vi "TL behavior P-Wall.vi"(1 "Behavior\nVelocity":dbl=20.0, 2 "Activate?":bool=TRUE, 3 "Sensor":T1=[{"Name"="bow", "Angle"=20.0, "Distance"=0.0}, {"Name"="pbow", "Angle"=60.0, "Distance"=0.0}, {"Name"="port", "Angle"=0.0, "Distance"=0.0}, {"Name"="sbow", "Angle"=60.0, "Distance"=0.0}, {"Name"="starboard", "Angle"=0.0, "Distance"=0.0}]) -> (0 "P-Wall Array":dbl[](array[numeric]))   [LabVIEW 2014]
doc: "This vi creates a array based upon the value of the PBow IR sensor reading."
uses:
  sensorsSTD.ctl
  <vilib>/addons/control/pid/pid.llb/PID (DBL).vi
  <vilib>/addons/control/pid/NI_PID_pid.lvlib
panel:
  in  "setpoint":dbl=40.0 format="%#_13g"
  out "steer":dbl format="%.2f"
  out "Sensor \nbeing used":string
  out "Waveform Graph":cluster{dbl, dbl, dbl[]}(graph)
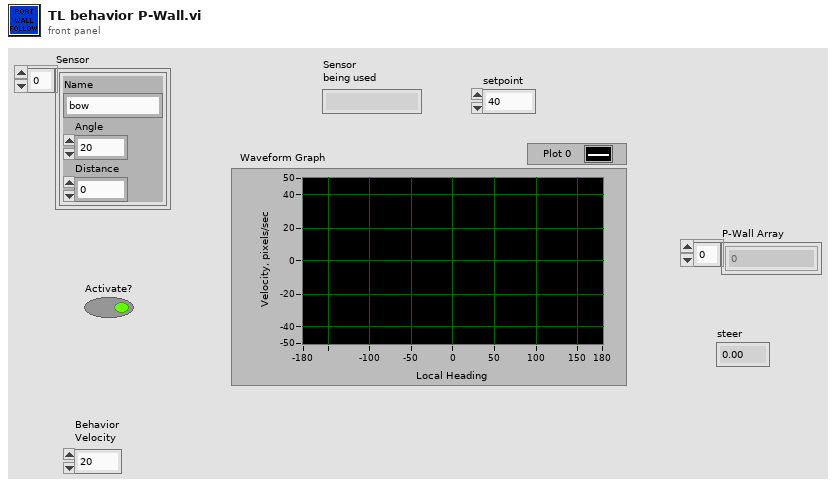
[diagram p1: front panel]
types:
  T1 = typedef "sensorsSTD.ctl" = cluster{"Name":string, "Angle":dbl, "Distance":dbl}[]
  T2 = cluster{"proportional gain (Kc)":dbl, "integral time (Ti, min)":dbl, "derivative time (Td, min)":dbl}
  T3 = cluster{"Name":string, "Angle":dbl, "Distance":dbl}
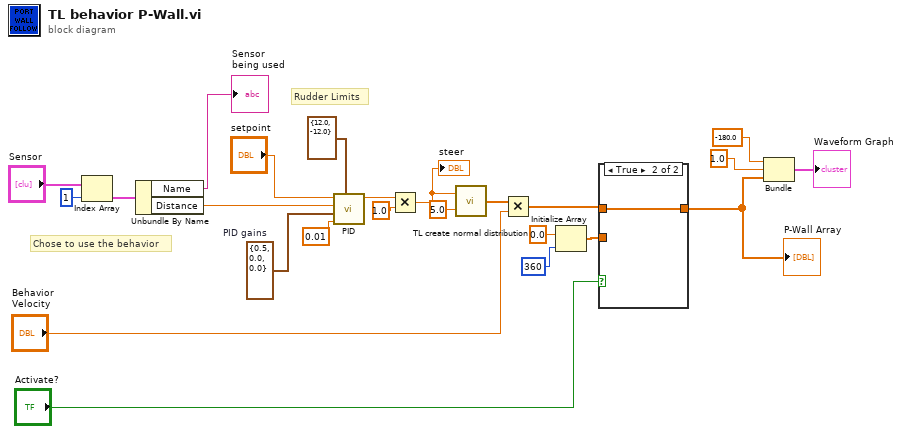
[diagram p0: block diagram]
diagram:
  w7 = T2 {"proportional gain (Kc)"=0.5, "integral time (Ti, min)"=0.0, "derivative time (Td, min)"=0.0}  # PID gains
  # "Rudder Limits"
  # "Chose to use the behavior"
  n1 = Index Array(array="Sensor", index=1) -> (element=w14:T3)
  n2 = Unbundle By Name(w14) -> ("Name"=→"Sensor \nbeing used":string, "Distance"=w6:dbl)
  n3 = call-poly <vilib>:"PID.vi"("output range"=cluster{"output high":dbl, "output low":dbl} {"output high"=12.0, "output low"=-12.0}, "dt (s)"=0.01, "PID gains"=w7, "process variable"=w6, "setpoint"="setpoint") -> ("output"=w11:dbl)  [unwired: 5 in, 1 out]
  n4 = Multiply(x=w11, y=1.0) -> (x*y=w5:dbl)
  "steer" <- w5
  n5 = call "TL create normal distribution.vi"("std (Normal)"=5.0, "mean"=w5) -> ("ACT array"=w4:dbl[])
  n6 = Multiply(x=w4, y="Behavior\nVelocity") -> (x*y=w3:dbl[])
  n7 = Initialize Array(0.0 ("element"), 360 ("dimension size")) -> (w18:dbl[])
  n8 = case shown="True" "Activate?" {
    tunnel: w18 -> [w25 _]
    tunnel: w3 -> [_ w26]
    tunnel: [w25 w26] -> w17
    frame False {
    }
    frame True {
    }
  }
  "P-Wall Array" <- w17
  n9 = Bundle(-180.0, 1.0, w17) -> (→"Waveform Graph":cluster{dbl, dbl, dbl[]})  [unwired: 1 in]
